vi "Set scintillator colors.vi"(8 "error in (no error)":errorcluster, 9 "Base alpha":sgl, 10 "Scintillators base color":u32(colorbox), 11 "Detector ref in":refnum<vi>) -> (0 "error out":errorcluster, 3 "Detector ref out":refnum<vi>)   [LabVIEW 2016]
uses:
  <vilib>/picture/3D Picture Control/NI_3D Picture Control.lvlib
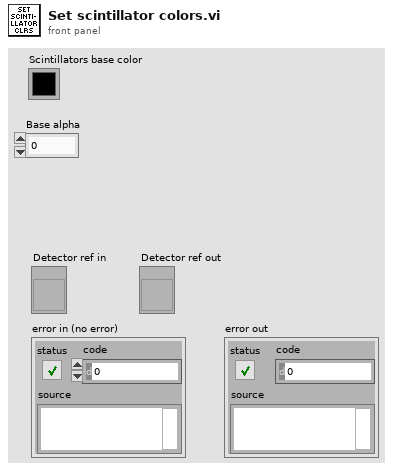
[diagram p1: front panel]
types:
  T1 = enum16{"Normal Bin", "Opaque Bin", "Transparent Bin"}
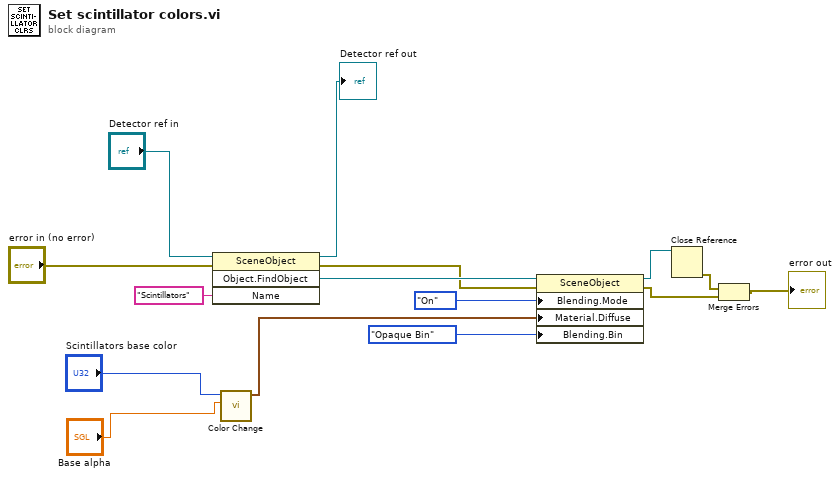
[diagram p0: block diagram]
diagram:
  n1 = invoke class="SceneObject" method="Object.FindObject"(reference="Detector ref in", error in="error in (no error)", "Name"="Scintillators") -> (reference out=→"Detector ref out":refnum<vi>, error out=w7:errorcluster, "FindObject"=w8:refnum<vi>)  [unwired: 1 in, 1 out]
  n2 = call <vilib>:"Color Change.vi"("Alpha"="Base alpha", "Color"="Scintillators base color") -> ("RGBA"=w2:cluster{"R":sgl, "G":sgl, "B":sgl, "A":sgl})  [unwired: 9 in]
  n3 = property class="SceneObject"(reference=w8, error in=w7, "Blending.Mode"=enum16{"Inherit Value", "Off", "On"}."On" ("Blending:Mode"), "Material.Diffuse"=w2, "Blending.Bin"=T1."Opaque Bin" ("Blending:Bin")) -> (reference out=w10:refnum<vi>, error out=w9:errorcluster)
  n4 = Close Reference(reference=w10) -> (error out=w11:errorcluster)  [unwired: 1 in]
  n5 = Merge Errors(w11, w9) -> (→"error out":errorcluster)
